vi "gc-zyklus mfc.vi"() -> ()   [LabVIEW 2010]
panel:
  out "Zeitpunkt":string
  out "Temperatur (°C)":u16
  out "Meßwert PC2 (mbara)":u16
  out "Meßwert PC1 (mbara)":u16
  out "Meßwert FC (mln/min)":u16
  in  "Setpoint PC1 (bara)":dbl min=0.15 max=3.0 step=0.05
  in  "Setpoint PC2 (bara)":dbl min=0.15 max=3.0 step=0.05
  in  "Dateipfad (Dialog verwenden)":path
  out "Zyklus Nr.":i32
  in  "Positionen (1-6)":i32[](array[numeric])=[1, 3, 5, 2]
  out "Anzahl der Zustände (Mpos.-Ventil)":i32
  out "Position":i32
  in  "Setpoints FC (ln/min)":dbl[](array[numeric])=[1.0, 3.0, 5.0, 2.0]
  in  "Längen der Zustände (s)":i32[](array[numeric])=[1, 3, 5, 2]
  out "Anzahl der Zustände (MFC)":i32
  out "Länge des Zustandes \"i\" (s)":i32
  out "Setpoint \"i\" FC (ln/min)":dbl
  out "Sequenz Nr.":i32
  out "Aktuelle Zeit":timestamp
  in  "(Sequenz wird zu Ende geführt)":bool
  # "Gerät im Chromatographie-Zyklus, z.B. MFC"
  # "Multipositionsventil"
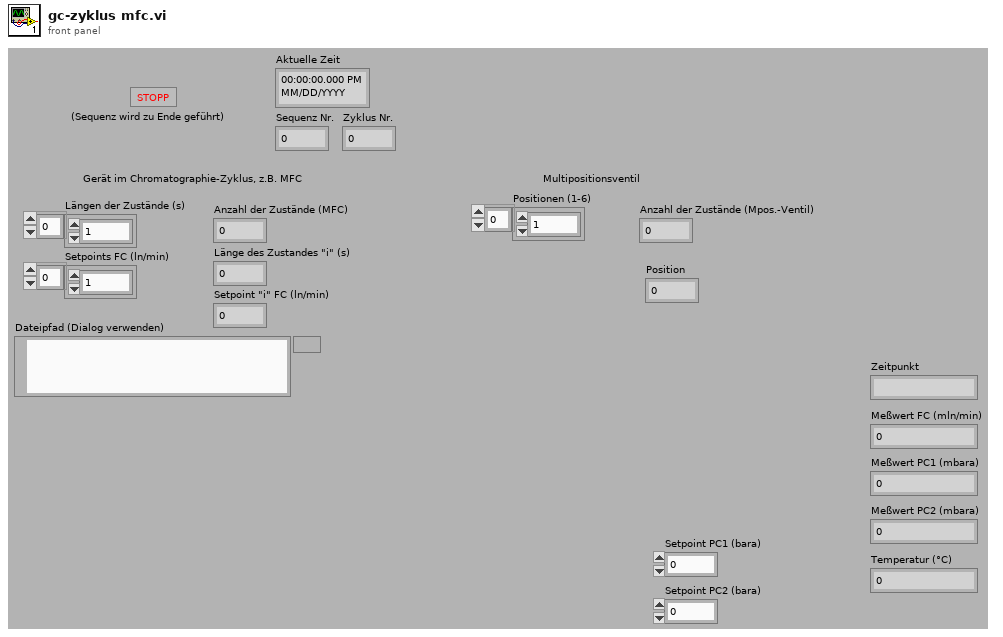
[diagram p1: front panel]
types:
  T1 = enum16{"open", "replace", "create", "open or create", "replace or create", "replace or create with confirmation"}
  T2 = cluster{"Mode":enum16{"RTU", "ASCII"}, "Slave Address":u8}
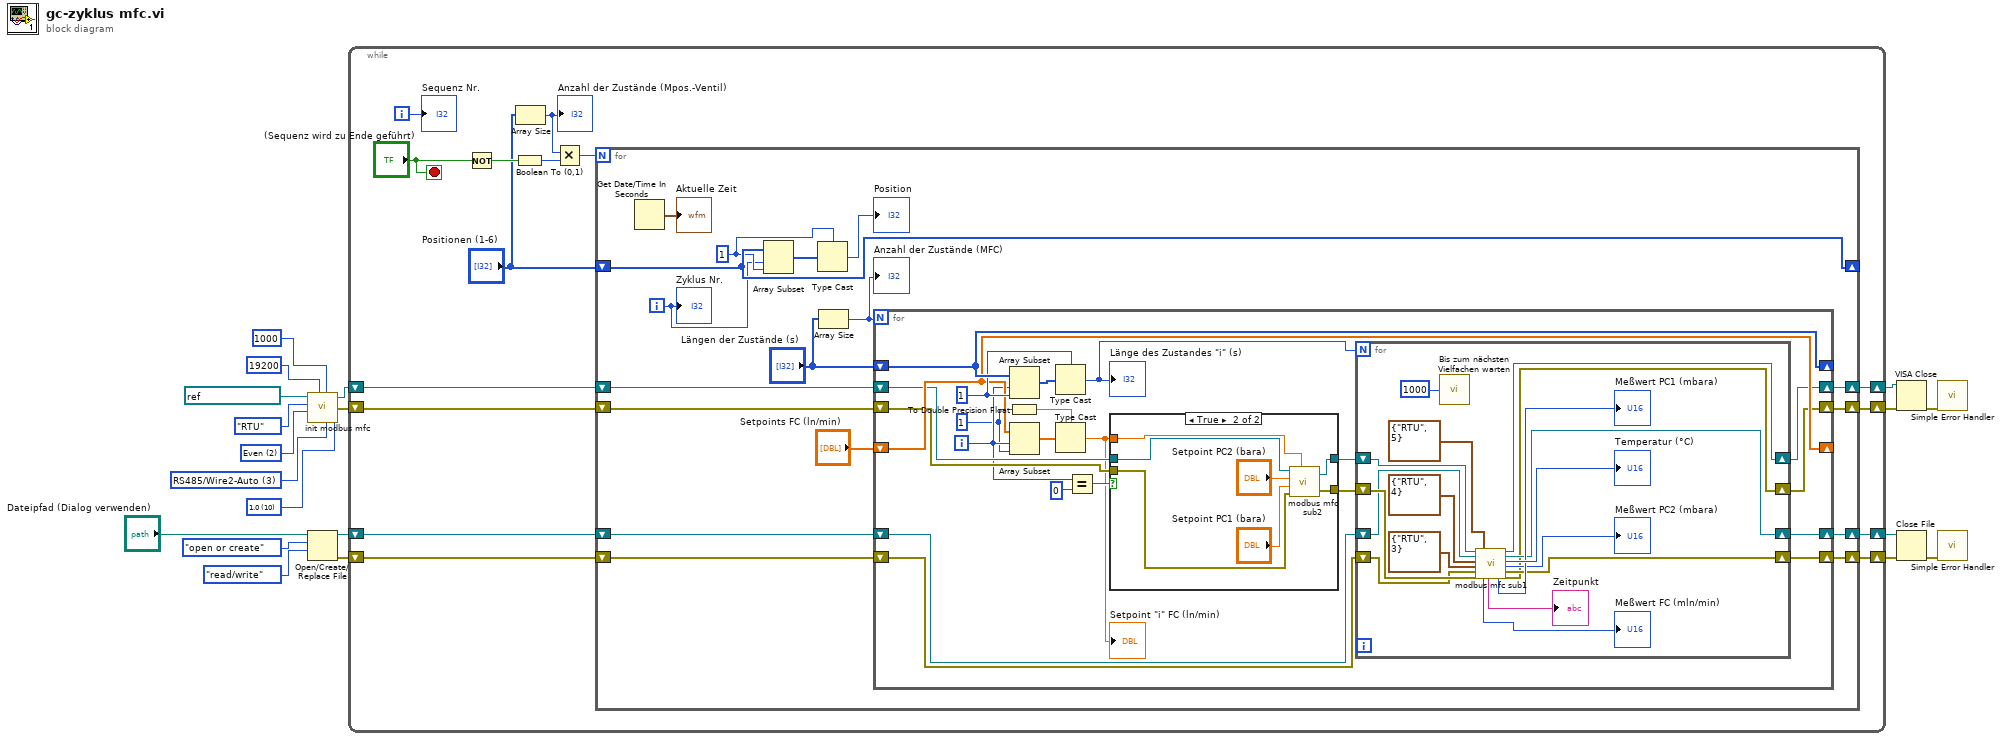
[diagram p0: block diagram]
diagram:
  w17 = u16 10 items=["1.0"=10, "1.5"=15, "2.0"=20] ("Serial Settings:Stop Bits")
  w15 = u16 2 items=["None", "Odd", "Even", "Mark", "Space"] ("Parity")
  w16 = i16 3 items=["Unknown"=-1, "RS485/Wire4"=0, "RS485/Wire2-EchoDTR"=1, "RS485/Wire2-CtrlDTR"=2, "RS485/Wire2-Auto"=3, "RS232/DTE"=128, "RS232/DCE"=129, "RS232/AUTO"=130] ("Serial Settings:Wire Mode")
  n1 = call "init modbus mfc.vi"("Timeout"=u32 1000, "Serial Settings:Stop Bits"=w17, "Serial Settings:Wire Mode"=w16, "Baud Rate"=u32 19200, "VISA resource name"=refnum<visa-resource-name> "ASRL2::INSTR", "Mode"=enum16{"RTU", "ASCII"}."RTU", "Parity"=w15) -> ("VISA resource name out"=w8:refnum<visa-resource-name>, "error out"=w7:errorcluster)  [unwired: 2 in]
  n2 = Open/Create/Replace File(file path (use dialog)="Dateipfad (Dialog verwenden)", operation (0:open)=T1."open or create" ("Operation (0:Öffnen)"), access (0:read/write)=enum16{"read/write", "read-only", "write-only"}."read/write" ("Zugriff (0:Lesen/Schreiben)")) -> (refnum out=w10:refnum<file>, error out=w9:errorcluster)  [unwired: 3 in, 1 out]
  n3 = while {
    shift-right: [w24] -> w4
    shift-left: w10 -> [w28]
    shift-right: [w23] -> w3
    shift-left: w9 -> [w27]
    shift-right: [w22] -> w2
    shift-left: w8 -> [w26]
    shift-right: [w21] -> w1
    shift-left: w7 -> [w25]
    i -> [w35]
    stop <- "(Sequenz wird zu Ende geführt)" stop-if-true
    n4 = Not(x="(Sequenz wird zu Ende geführt)") -> (.not. x?=w32:bool)
    n5 = Boolean To (0,1)(Boolean=w32) -> (0, 1=w30:i16)
    n6 = Array Size(array="Positionen (1-6)") -> (size(s)=w34:i32)
    "Anzahl der Zustände (Mpos.-Ventil)" <- w34
    n7 = Multiply(x=w34, y=w30) -> (x*y=w31:i32)
    n8 = for {
      N: w31 -> [_]
      shift-right: [w52] -> _
      shift-left: "Positionen (1-6)" -> [w52]
      shift-right: [w40] -> w24
      shift-left: w28 -> [w41]
      shift-right: [w38] -> w23
      shift-left: w27 -> [w42]
      shift-right: [w39] -> w22
      shift-left: w26 -> [w44]
      shift-right: [w37] -> w21
      shift-left: w25 -> [w43]
      i -> [w48]
      w51 = 1 ("Länge")
      n9 = Get Date/Time In Seconds() -> (seconds since 1Jan1904=→"Aktuelle Zeit":timestamp)
      n10 = Array Subset(array=w52, index=w48, length=w51) -> (w50:i32[])
      n11 = Type Cast(type=w51, x=w50) -> (*(type *) &x=→"Position":i32)
      n12 = Array Size(array="Längen der Zustände (s)") -> (size(s)=w36:i32)
      "Anzahl der Zustände (MFC)" <- w36
      n13 = for {
        N: w36 -> [_]
        shift-right: [w74] -> _
        shift-left: "Längen der Zustände (s)" -> [w74]
        shift-right: [w70] -> _
        shift-left: "Setpoints FC (ln/min)" -> [w70]
        shift-right: [w57] -> w40
        shift-left: w41 -> [w58]
        shift-right: [w55] -> w38
        shift-left: w42 -> [w59]
        shift-right: [w56] -> w39
        shift-left: w44 -> [w69]
        shift-right: [w54] -> w37
        shift-left: w43 -> [w68]
        i -> [w67]
        w63 = 1 ("Länge")
        w73 = 1 ("Länge")
        n14 = Array Subset(array=w74, index=w67, length=w73) -> (w72:i32[])
        n15 = To Double Precision Float(number=w63) -> (double precision float=w62:dbl)
        n16 = Array Subset(array=w70, index=w67, length=w63) -> (w71:dbl[])
        n17 = Type Cast(type=w73, x=w72) -> (*(type *) &x=w64:i32)
        "Länge des Zustandes \"i\" (s)" <- w64
        n18 = Type Cast(type=w62, x=w71) -> (*(type *) &x=w53:dbl)
        "Setpoint \"i\" FC (ln/min)" <- w53
        n19 = Equal?(x=w67, y=0) -> (x = y?=w65:bool)
        n20 = case shown="True" w65 {
          tunnel: w68 -> [w93 w99]
          tunnel: [w93 w98] -> w61
          tunnel: w69 -> [w92 w100]
          tunnel: [w92 w97] -> w60
          tunnel: w53 -> [_ w94]
          frame False {
          }
          frame True {
            n21 = call "modbus mfc sub2.vi"("VISA resource name out 2"=w100, "Setpoint PC2 (bara)"="Setpoint PC2 (bara)", "Setpoint PC1 (bara)"="Setpoint PC1 (bara)", "error out 2"=w99, "Setpoint FC (ln/min)"=w94) -> ("VISA resource name out"=w97:refnum<visa-resource-name>, "error out"=w98:errorcluster)
          }
        }
        n22 = for {
          N: w64 -> [_]
          shift-right: [w77] -> w56
          shift-left: w60 -> [w81]
          shift-right: [w78] -> w57
          shift-left: w58 -> [w79]
          shift-right: [w76] -> w55
          shift-left: w59 -> [w80]
          shift-right: [w75] -> w54
          shift-left: w61 -> [w82]
          n23 = call "Bis zum nächsten Vielfachen warten"("Count(mSec)"=u32 1000) -> ()  [unwired: 1 out]
          n24 = call "modbus mfc sub1.vi"("VISA resource name out"=w81, "refnum out 2"=w79, "Serial Parameters 2"=T2 {"Mode"=enum."RTU", "Slave Address"=4}, "Serial Parameters"=T2 {"Mode"=enum."RTU", "Slave Address"=3}, "error out 2"=w80, "error out 3"=w82, "Serial Parameters 3"=T2 {"Mode"=enum."RTU", "Slave Address"=5}) -> ("Numerisch 3"=→"Meßwert FC (mln/min)":u16, "date/time string"=→"Zeitpunkt":string, "Numerisch 2"=→"Meßwert PC1 (mbara)":u16, "VISA resource name out 2"=w77:refnum<visa-resource-name>, "refnum out"=w78:refnum<file>, "Numerisch 4"=→"Temperatur (°C)":u16, "Numerisch"=→"Meßwert PC2 (mbara)":u16, "error out"=w76:errorcluster, "error out 4"=w75:errorcluster)  [unwired: 3 in, 1 out]
        }
      }
      "Zyklus Nr." <- w48
    }
    "Sequenz Nr." <- w35
  }
  n25 = VISA Close(VISA resource name=w2, error in (no error)=w1) -> (error out=w6:errorcluster)
  n26 = Close File(refnum=w4, error in=w3) -> (error out=w5:errorcluster)  [unwired: 1 out]
  n27 = call <vilib>:"Simple Error Handler.vi"("error in (no error)"=w6) -> ()  [unwired: 4 in, 5 out]
  n28 = call <vilib>:"Simple Error Handler.vi"("error in (no error)"=w5) -> ()  [unwired: 4 in, 5 out]
